vi "init classes.vi"(6 "SP timeouts":T1={"reconn_timeout"=30000, "read_timeout"=50, "N attempt max"=3, "t_reset_TTL"=120000, "period"=10000} {"read_timeout" min=1 max=5000 step=1; "t_reset_TTL" min=10 max=100000 step=1; "period" min=10 max=100000 step=1; "N attempt max" min=10 max=240000 step=1; "reconn_timeout" min=10 max=240000 step=1}, 8 "error in (no error)":errorcluster, 9 "conninfo":T2, 10 "object name":string="AA1", 11 "Status":T3) -> (0 "error out":errorcluster, 3 "classes":refnum<class "Save messages PGserver.lvclass">[](array[class]))   [LabVIEW 2019, in "PostgreSQL.lvlib"]
uses:
  PostgreSQL.lvlib
  Save messages PGserver/Save messages PGserver.lvclass
  Modbus/Eth Status/Ctl/Status.ctl
  Modbus/MB_TCP2/MB_TCP_State.ctl
  ctl/Coninfo.ctl
  ctl/Save_prog_timeouts.ctl
  PG analogs/PG analogs.lvclass
  D:/my_projects/projects/Algorithms/Labview/19/Database/Save messages PGserver/Save messages PGserver.lvclass
  PG messages/PG messages.lvclass
  PG alarms/PG alarms.lvclass
  Save messages PGserver/Save messages PGserver.lvclass/Save messages PGserver.ctl
  Modbus/MB_TCP2/MB_TCP.lvclass
  Modbus/Eth Status/Eth Status.lvlib
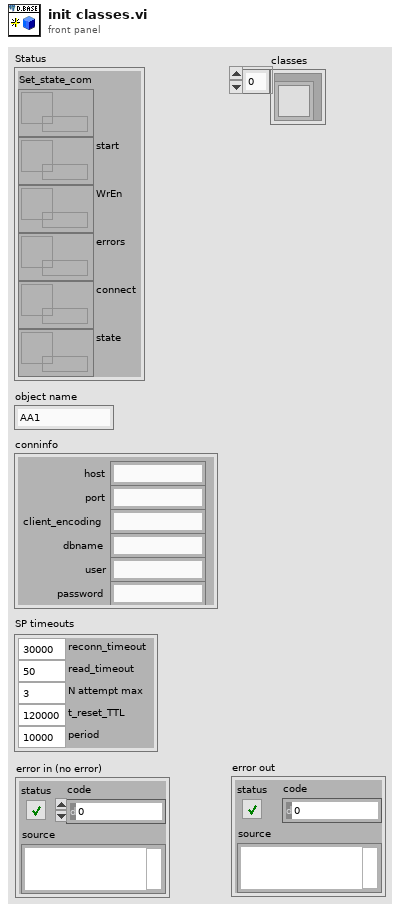
[diagram p1: front panel]
types:
  T1 = typedef "PostgreSQL.lvlib/Save_prog_timeouts.ctl" = cluster{"reconn_timeout":i32, "read_timeout":i32, "N attempt max":i32, "t_reset_TTL":i32, "period":i32}
  T2 = typedef "PostgreSQL.lvlib/Coninfo.ctl" = cluster{"host":string, "port":string, "client_encoding":string, "dbname":string, "user":string, "password":string}
  T3 = typedef "Eth Status.lvlib/Status.ctl" = cluster{"Set_state_com":refnum<data-value>, "start":refnum<data-value>, "WrEn":refnum<data-value>, "errors":refnum<data-value>, "connect":refnum<data-value>, "state":refnum<data-value>}
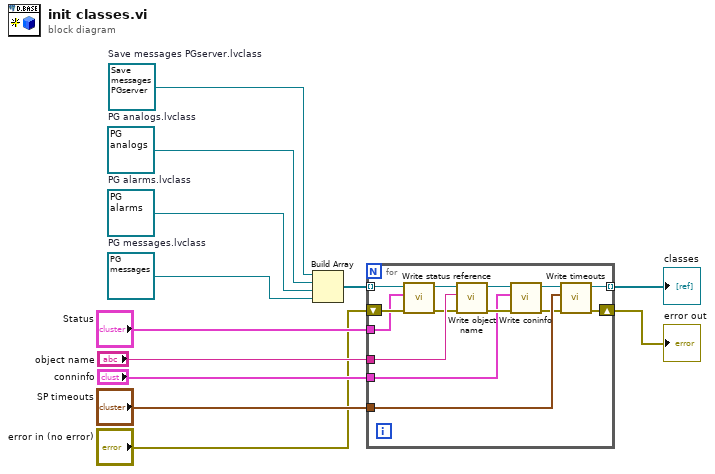
[diagram p0: block diagram]
diagram:
  w9 = refnum<class "PG analogs.lvclass"> refnum  # PG analogs.lvclass
  w11 = refnum<class "PG messages.lvclass"> refnum  # PG messages.lvclass
  w10 = refnum<class "PG alarms.lvclass"> refnum  # PG alarms.lvclass
  w12 = refnum<class "Save messages PGserver.lvclass"> refnum  # Save messages PGserver.lvclass
  n1 = Build Array(w12, w9, w10, w11) -> (w8:refnum<class "Save messages PGserver.lvclass">[])
  n2 = for {
    tunnel: w8 -> [w22] mode=indexing
    tunnel: "object name" -> [w26]
    shift-right: [w14] -> w1
    shift-left: "error in (no error)" -> [w20]
    tunnel: "conninfo" -> [w23]
    tunnel: "Status" -> [w18]
    tunnel: "SP timeouts" -> [w17]
    tunnel: [w13] -> w7 mode=indexing
    n3 = call "Write status reference.vi"("error in (no error)"=w20, "Status"=w18, "SP in"=w22) -> ("error out"=w19:errorcluster, "SP out"=w21:refnum<class "Save messages PGserver.lvclass">)  [unwired: 7 in]
    n4 = call "Write object name.vi"("error in (no error)"=w19, "object name"=w26, "SP in"=w21) -> ("error out"=w24:errorcluster, "SP out"=w25:refnum<class "Save messages PGserver.lvclass">)  [unwired: 7 in]
    n5 = call "Write coninfo.vi"("error in (no error)"=w24, "conninfo"=w23, "SP in"=w25) -> ("error out"=w15:errorcluster, "SP out"=w16:refnum<class "Save messages PGserver.lvclass">)  [unwired: 7 in]
    n6 = call "Write timeouts.vi"("error in (no error)"=w15, "SP timeouts"=w17, "SP in"=w16) -> ("error out"=w14:errorcluster, "SP out"=w13:refnum<class "Save messages PGserver.lvclass">)  [unwired: 7 in]
  }
  "classes" <- w7
  "error out" <- w1
